vi "Release UDP Handle.vi"(8 "error in (no error)":errorcluster, 11 "PF_API in":refnum<class "PF_API.lvclass">) -> (0 "error out":errorcluster, 3 "PF_API out":refnum<class "PF_API.lvclass">)   [LabVIEW 2019, in "PF_API.lvclass"]
doc: "Finishes the UDP connection on both scanner and host."
uses:
  PF_API.lvclass
  PF_API.lvclass/PF_API.ctl
  <vilib>/httpClient/POSTBuffer.vi
  <vilib>/httpClient/LabVIEWHTTPClient.lvlib
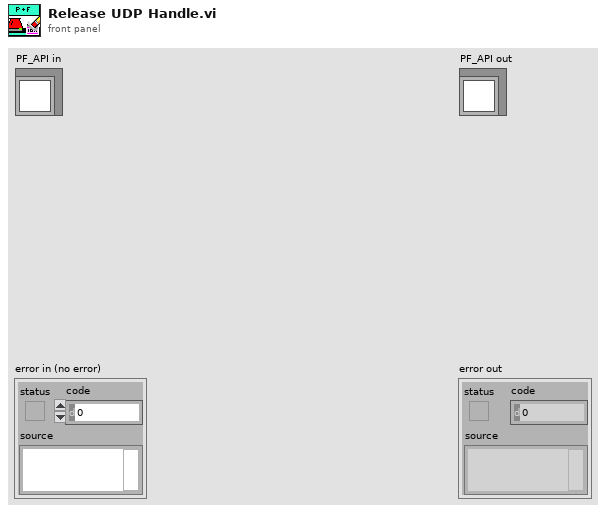
[diagram p1: front panel]
types:
  T1 = typedef "LabVIEWHTTPClient.lvlib/ClientHandle.ctl" = refnum<k1>
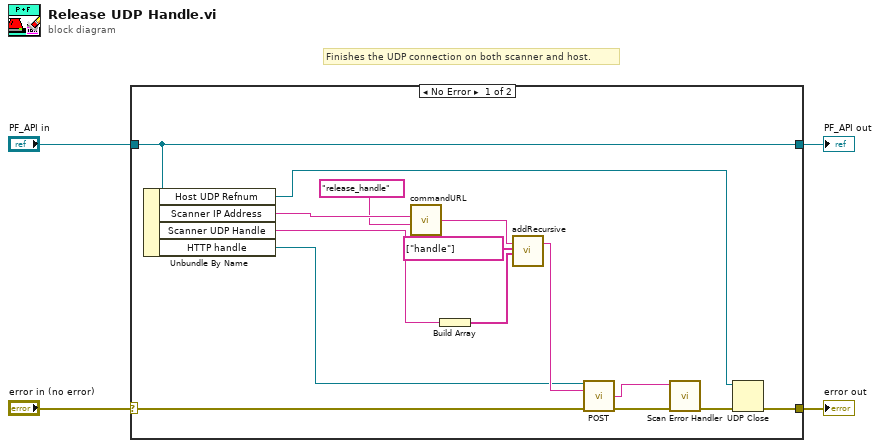
[diagram p0: block diagram]
diagram:
  # "Finishes the UDP connection on both scanner and host."
  n1 = case shown="No Error" "error in (no error)" {
    selector: "error in (no error)" -> [w19 w21]
    tunnel: [w6 w21] -> w3
    tunnel: [w18 w20] -> w1
    tunnel: "PF_API in" -> [w18 w20]
    frame No Error {
      n2 = Unbundle By Name(w18) -> ("Host UDP Refnum"=w5:refnum<k16>, "Scanner IP Address"=w16:string, "Scanner UDP Handle"=w12:string, "HTTP handle"=w9:T1)
      n3 = call "commandURL.vi"("Command String"="release_handle", "Scanner IP Address"=w16) -> ("Command URL"=w14:string)  [unwired: 4 in]
      n4 = Build Array(w12) -> (w11:string[])
      n5 = call "addRecursive.vi"("Command URL in"=w14, "Parameter Key"=string[] ["handle"], "Parameter Value"=w11) -> ("Command URL out"=w10:string)  [unwired: 13 in, 3 out]
      n6 = call-poly <vilib>:"POST.vi"("client handle"=w9, "url"=w10, "error in (no error)"=w19) -> ("body"=w7:string, "error out"=w17:errorcluster)  [unwired: 9 in, 2 out]
      n7 = call "Scan Error Handler.vi"("Error In"=w17, "HTTP Response"=w7) -> ("Error Out"=w8:errorcluster)  [unwired: 9 in]
      n8 = UDP Close(connection ID=w5, 8:w8) -> (error out=w6:errorcluster)  [unwired: 1 out]
    }
    frame Error {
    }
  }
  "error out" <- w3
  "PF_API out" <- w1
